vi "Toggle With Reset.vi"(1 "Reset":bool, 2 "Boolean":bool) -> (0 "Driver Switch 2":bool)   [LabVIEW 2015]
doc: "This VI takes a Boolean Value which once it turns from true to false it stores a true value for Driver Switch 2 (the output) until either the Reset value is true or the Boolean value is turned from true to false again. An example of implementing this would be a claw which can be opened or closed with a button but also can be closed if a limit switch on the claw is engaged (i.e there is something in the claw)."
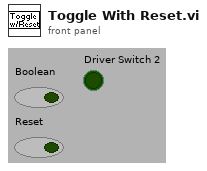
[diagram p1: front panel]
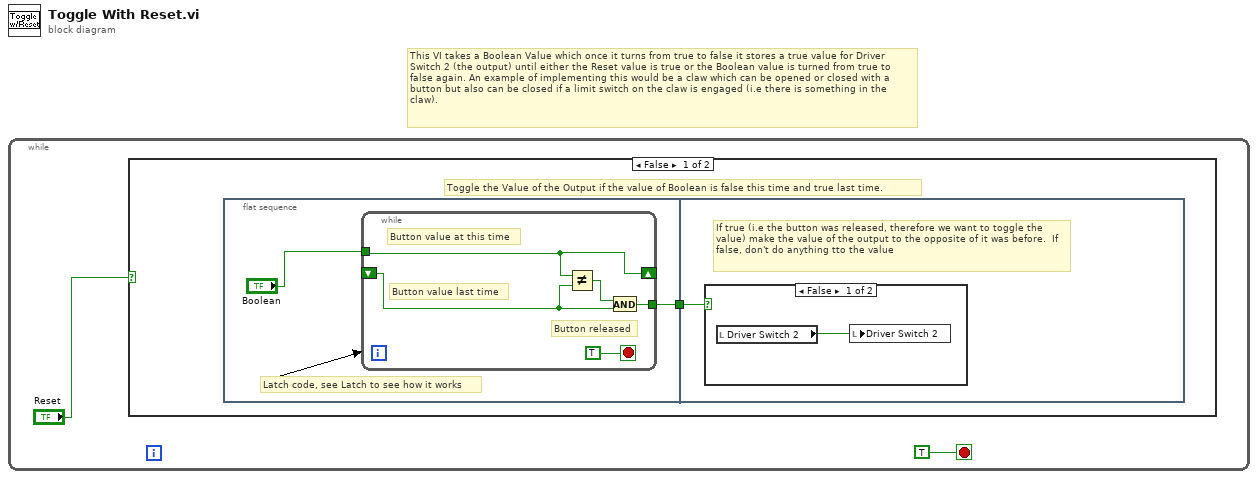
[diagram p0: block diagram]
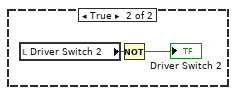
[diagram p2: hidden frame]
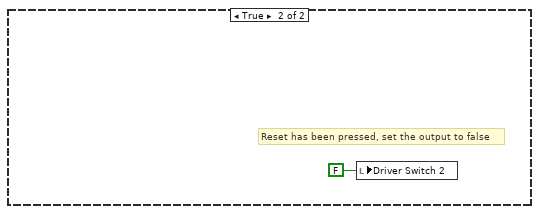
[diagram p3: hidden frame]
diagram:
  # "This VI takes a Boolean Value which once it turns from true to false it stores a true value for Driver Switch 2 (the output) until either the Reset value is true or the Boolean value is turned from true to false again. An example of implementing this would be a claw which can be opened or closed with a button but also can be closed if a limit switch on the claw is engaged (i.e there is something in the claw)."
  n1 = while {
    stop <- TRUE stop-if-true
    n2 = case shown="False" "Reset" {
      frame False {
        # "Toggle the Value of the Output if the value of Boolean is false this time and true last time."
        n3 = flat-sequence {
          tunnel: [w4] -> w3
          tunnel: w3 -> [w11]
          frame #0 {
            # "Latch code, see Latch to see how it works"
            n4 = while {
              tunnel: [w9] -> w4
              tunnel: "Boolean" -> [w8]
              shift-right: [w8] -> _
              shift-left: _ -> [w7]
              stop <- TRUE ("stop") stop-if-true
              # "Button released"
              # "Button value last time"
              # "Button value at this time"
              n5 = Not Equal?(x=w8, y=w7) -> (x != y?=w10:bool)
              n6 = And(x=w10, y=w7) -> (x .and. y?=w9:bool)
            }
          }
          frame #1 {
            # "If true (i.e the button was released, therefore we want to toggle the value) make the value of the output to the opposite of it was before.  If false, don't do anything tto the value"
            n7 = case shown="False" w11 {
              frame False {
                n8 = local read "Driver Switch 2"() -> (w12:bool)
                n9 = local write "Driver Switch 2"(w12) -> ()
              }
              frame True {
                n10 = local read "Driver Switch 2"() -> (w14:bool)
                n11 = Not(x=w14) -> (.not. x?=→"Driver Switch 2":bool)
              }
            }
          }
        }
      }
      frame True {
        # "Reset has been pressed, set the output to false"
        n12 = local write "Driver Switch 2"(FALSE ("Driver Switch 2")) -> ()
      }
    }
  }
